vi "transmitter1.vi"() -> ()   [LabVIEW 2013]
uses:
  <vilib>/sound2/lvsound2.llb/Sound File Info (path).vi
  <vilib>/sound2/lvsound2.llb/Sound File Read Open.vi
  <vilib>/Analysis/2dsp.llb/Rational Resample (single channel, DBL).vi
  <vilib>/sound2/lvsound2.llb/Sound File Read (DBL).vi
  <instrlib>/niUSRP/niUSRP Write Tx Data (CDB).vi
  <vilib>/Analysis/NI_AALPro.lvlib
panel:
  out "Constellation":cluster{dbl[], dbl[]}(graph)
  in  "FM deviation (Hz)":dbl=100000.0 format="%#_6p"
  out "output Waveform":waveform(dbl)(graph)
  in  "number of samples":i32=-1
  in  "path":path
  out "error out":errorcluster
  out "coerced gain":dbl format="%#_6f"
  out "coerced carrier frequency":dbl=100000.0 format="%#_6p"
  out "coerced IQ rate":dbl=100000.0 format="%#_6p"
  in  "stop":bool
  in  "active antenna":string
  in  "gain":dbl format="%#_6f"
  in  "carrier frequency":dbl=100000.0 format="%#_6p"
  in  "IQ rate":dbl=100000.0 format="%#_6p"
  in  "device names":refnum<k15>
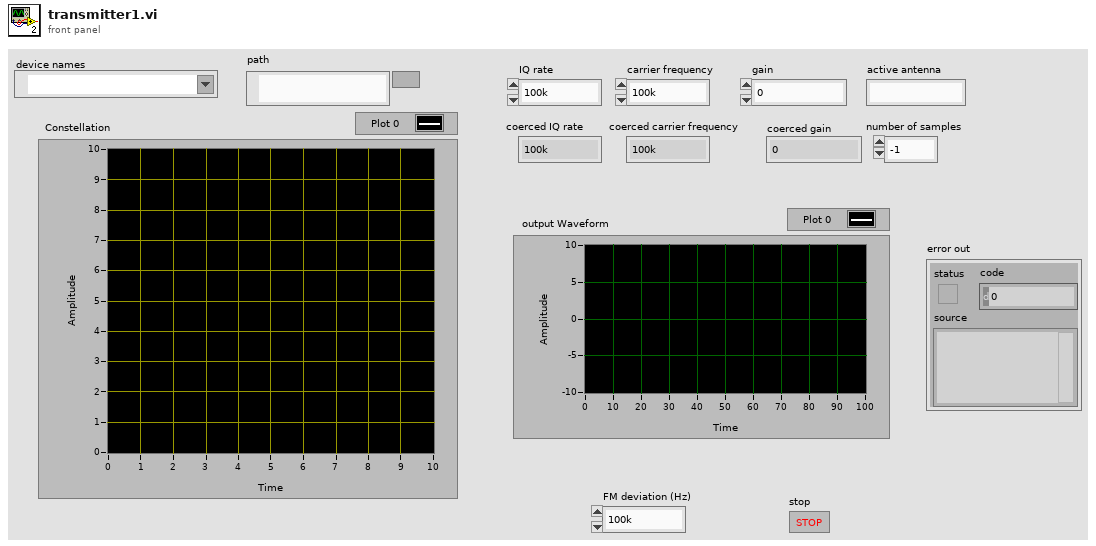
[diagram p1: front panel]
types:
  T1 = typedef "Sound Data Format.ctl" = cluster{"sample rate (S/s)":dbl, "number of channels":i32, "bits per sample":i32}
  T2 = typedef "Sound File Refnum.ctl" = refnum<file>
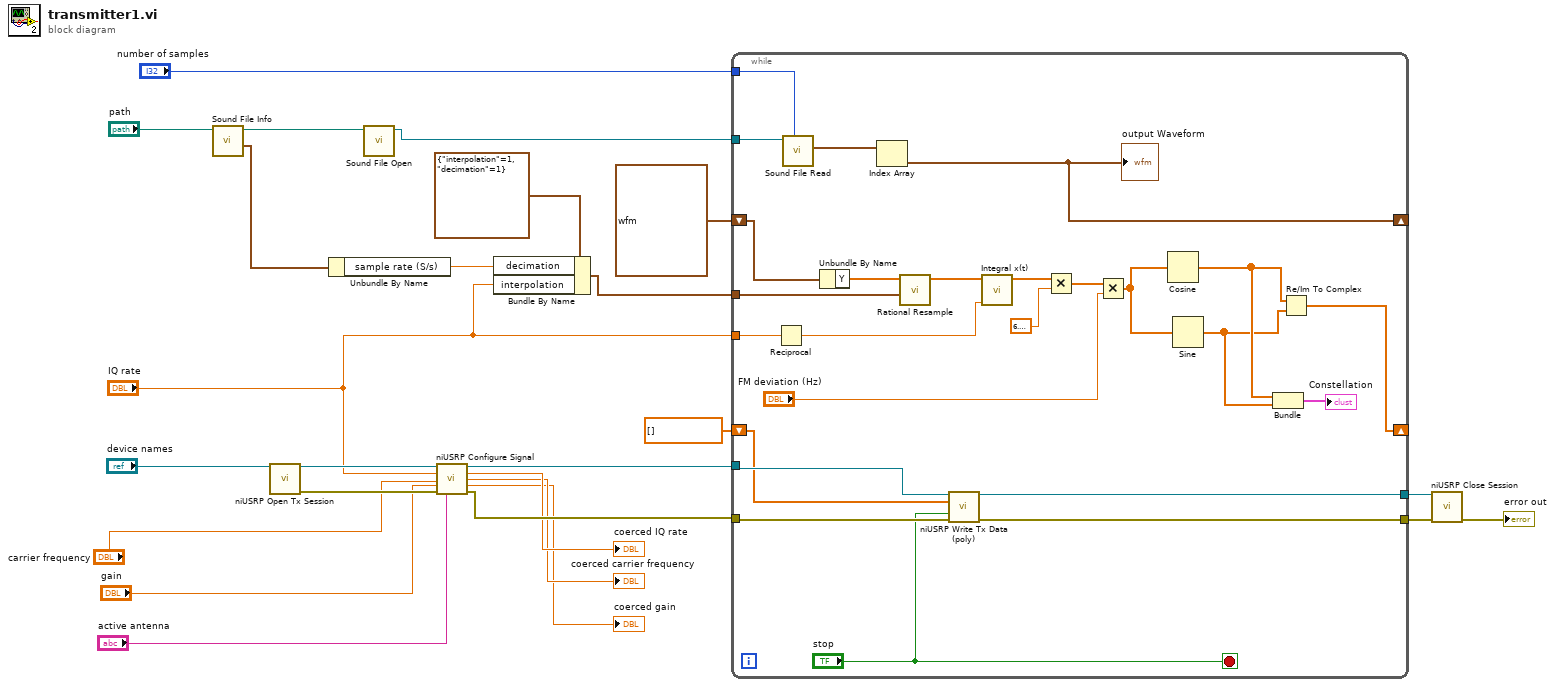
[diagram p0: block diagram]
diagram:
  n1 = call-poly <vilib>:"Sound File Info.vi"("path"="path") -> ("sound format"=w7:T1, "path out"=w10:path)  [unwired: 7 in, 2 out]
  n2 = call <instrlib>:"niUSRP Open Tx Session.vi"("device names"="device names") -> ("session handle out"=w24:refnum<k15>, "error out"=w23:errorcluster)  [unwired: 13 in]
  n3 = Unbundle By Name(w7) -> ("sample rate (S/s)"=w3:dbl)
  n4 = call-poly <vilib>:"Sound File Open.vi"("path"=w10) -> ("sound file refnum"=w8:T2)  [unwired: 9 in, 1 out]
  n5 = call <instrlib>:"niUSRP Configure Signal.vi"("session handle"=w24, "IQ rate"="IQ rate", "carrier frequency"="carrier frequency", "gain"="gain", "error in (no error)"=w23, "active antenna"="active antenna") -> ("session handle out"=w19:refnum<k15>, "coerced IQ rate"=→"coerced IQ rate":dbl, "coerced carrier frequency"=→"coerced carrier frequency":dbl, "coerced gain"=→"coerced gain":dbl, "error out"=w18:errorcluster)  [unwired: 5 in]
  n6 = Bundle By Name(cluster=cluster{"interpolation":i32, "decimation":i32} {"interpolation"=1, "decimation"=1} ("input cluster"), "decimation"=w3, "interpolation"="IQ rate") -> (w2:cluster{"interpolation":i32, "decimation":i32})
  n7 = while {
    tunnel: w19 -> [w50]
    tunnel: w18 -> [w49]
    tunnel: [w48] -> w14
    tunnel: [w47] -> w13
    tunnel: "number of samples" -> [w45]
    tunnel: w8 -> [w44]
    shift-right: [w42] -> _
    shift-left: waveform(dbl) {"t0"=timestamp(0 s since 1904-01-01), "dt"=1.0, "Y"=[]} ("data") -> [w41]
    tunnel: "IQ rate" -> [w37]
    shift-right: [w29] -> _
    shift-left: cdb[] [] -> [w27]
    tunnel: w2 -> [w28]
    stop <- "stop" stop-if-true
    n8 = Reciprocal(x=w37) -> (1/x=w38:dbl)
    n9 = call-poly <vilib>:"Sound File Read.vi"("number of samples/ch (-1: all)"=w45, "sound file refnum"=w44) -> ("data"=w43:waveform(dbl)[])  [unwired: 5 in, 4 out]
    n10 = Unbundle By Name(w41) -> ("Y"=w40:dbl[])
    n11 = Index Array(array=w43) -> (element=w42:waveform(dbl))  [unwired: 1 in]
    "output Waveform" <- w42
    n12 = call-poly <vilib>:"Rational Resample.vi"("resample factor"=w28, "X"=w40) -> ("Y"=w39:dbl[])  [unwired: 7 in, 2 out]
    n13 = call-poly <instrlib>:"niUSRP Write Tx Data (poly).vi"("session handle"=w50, "data"=w27, "end of data?"="stop", "error in (no error)"=w49) -> ("session handle out"=w48:refnum<k15>, "error out"=w47:errorcluster)  [unwired: 10 in]
    n14 = call <vilib>:"Integral x(t).vi"("dt"=w38, "X"=w39) -> ("Integral X"=w35:dbl[])  [unwired: 8 in, 1 out]
    n15 = Multiply(x=w35, y=6.283185307179586) -> (x*y=w34:dbl[])
    n16 = Multiply(x=w34, y="FM deviation (Hz)") -> (x*y=w33:dbl[])
    n17 = Cosine(x=w33) -> (cos(x)=w31:dbl[])
    n18 = Sine(x=w33) -> (sin(x)=w30:dbl[])
    n19 = Bundle(w31, w30) -> (→"Constellation":cluster{dbl[], dbl[]})  [unwired: 1 in]
    n20 = Re/Im To Complex(1:w30, 2:w31) -> (0:w29:cdb[])
  }
  n21 = call <instrlib>:"niUSRP Close Session.vi"("session handle"=w14, "error in (no error)"=w13) -> ("error out"=→"error out":errorcluster)  [unwired: 13 in]
